vi "Test Set Subpanels-- Paths Array.vi"(8 "error in":errorcluster) -> (0 "error out":errorcluster)   [LabVIEW 2020]
uses:
  Maui 2.0/Maui 2.0.lvclass
  C:/Program Files (x86)/National Instruments/LabVIEW 2020/vi.lib/JKI/JKI SMO/SMO/SMO.lvclass
  <vilib>/addons/_JKI Toolkits/Caraya/classes/Assert/Assert True.vi
  <vilib>/JKI/JKI SMO/SMO/SMO.lvclass
  <vilib>/addons/_JKI Toolkits/Caraya/classes/Test/Test.lvclass
  <vilib>/addons/_JKI Toolkits/Caraya/classes/Assert/Assert.lvclass
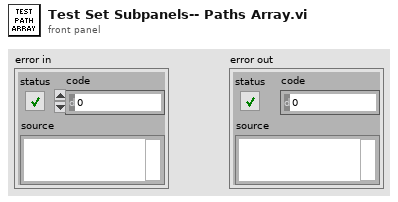
[diagram p1: front panel]
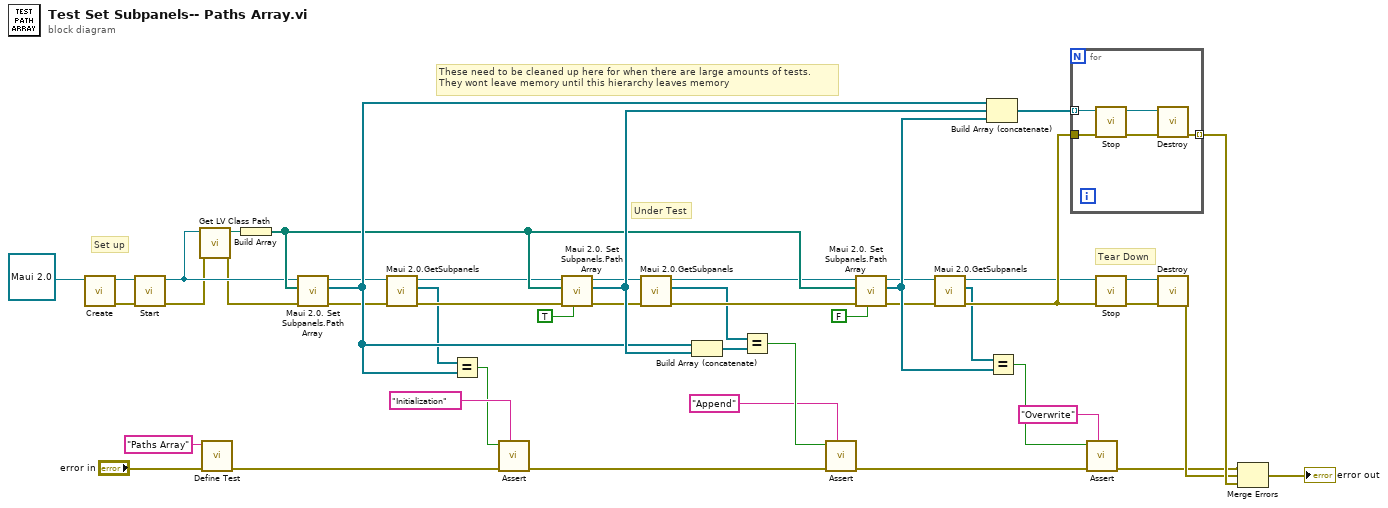
[diagram p0: block diagram]
diagram:
  # "These need to be cleaned up here for when there are large amounts of tests.\nThey wont leave memory until this hierarchy leaves memory"
  # "Tear Down"
  # "Set up"
  # "Under Test"
  n1 = call <vilib>:"Create.vi"("SMO"=refnum<class "Maui 2.0.lvclass"> refnum ("Maui 2.0.lvclass")) -> ("error out"=w3:errorcluster, "SMO out"=w2:refnum<class "Maui 2.0.lvclass">)  [unwired: 8 in, 1 out]
  n2 = call <vilib>:"Start.vi"("error in (no error)"=w3, "SMO"=w2) -> ("error out"=w13:errorcluster, "SMO out"=w15:refnum<class "Maui 2.0.lvclass">)  [unwired: 8 in]
  n3 = call <vilib>:"Get LV Class Path.vi"("error in (no error)"=w13, "object"=w15) -> ("error out"=w14:errorcluster, "class path"=w12:path)  [unwired: 8 in]
  n4 = call <vilib>:"Define Test.vi"("error in (no error)"="error in", "Label (VI Title)"="Paths Array") -> ("error out"=w41:errorcluster)  [unwired: 9 in]
  n5 = Build Array(w12) -> (w31:path[])
  n6 = call-dynamic "Maui 2.0. Set Subpanels.Path Array.vi"("error in (no error)"=w14, "Subpanel List"=w31, "Maui 2.0 in"=w15) -> ("error out"=w5:errorcluster, "Subpanels"=w42:refnum<class "SMO.lvclass">[], "Maui 2.0 out"=w4:refnum<class "Maui 2.0.lvclass">)  [unwired: 6 in]
  n7 = call "Maui 2.0.GetSubpanels.vi"("error in (no error)"=w5, "Maui 2.0"=w4) -> ("error out"=w18:errorcluster, "Subpanels"=w6:refnum<class "SMO.lvclass">[], "Maui 2.0 out"=w17:refnum<class "Maui 2.0.lvclass">)  [unwired: 7 in]
  n8 = Equal?(x=w6, y=w42) -> (x = y?=w10:bool)
  n9 = call-poly <vilib>:"Assert.vi"("Label"="Initialization", "error in (no error)"=w41, "True?"=w10) -> ("error out"=w33:errorcluster)  [unwired: 8 in]
  n10 = call-dynamic "Maui 2.0. Set Subpanels.Path Array.vi"("Append (F)"=TRUE, "error in (no error)"=w18, "Subpanel List"=w31, "Maui 2.0 in"=w17) -> ("error out"=w20:errorcluster, "Subpanels"=w43:refnum<class "SMO.lvclass">[], "Maui 2.0 out"=w19:refnum<class "Maui 2.0.lvclass">)  [unwired: 5 in]
  n11 = call "Maui 2.0.GetSubpanels.vi"("error in (no error)"=w20, "Maui 2.0"=w19) -> ("error out"=w30:errorcluster, "Subpanels"=w21:refnum<class "SMO.lvclass">[], "Maui 2.0 out"=w28:refnum<class "Maui 2.0.lvclass">)  [unwired: 7 in]
  n12 = Build Array (concatenate)(w42, w43) -> (w22:refnum<class "SMO.lvclass">[])
  n13 = Equal?(x=w21, y=w22) -> (x = y?=w25:bool)
  n14 = call-poly <vilib>:"Assert.vi"("Label"="Append", "error in (no error)"=w33, "True?"=w25) -> ("error out"=w34:errorcluster)  [unwired: 8 in]
  n15 = call-dynamic "Maui 2.0. Set Subpanels.Path Array.vi"("Append (F)"=FALSE, "error in (no error)"=w30, "Subpanel List"=w31, "Maui 2.0 in"=w28) -> ("error out"=w26:errorcluster, "Subpanels"=w44:refnum<class "SMO.lvclass">[], "Maui 2.0 out"=w27:refnum<class "Maui 2.0.lvclass">)  [unwired: 5 in]
  n16 = call "Maui 2.0.GetSubpanels.vi"("error in (no error)"=w26, "Maui 2.0"=w27) -> ("error out"=w46:errorcluster, "Subpanels"=w35:refnum<class "SMO.lvclass">[], "Maui 2.0 out"=w29:refnum<class "Maui 2.0.lvclass">)  [unwired: 7 in]
  n17 = Build Array (concatenate)(w42, w43, w44) -> (w45:refnum<class "SMO.lvclass">[])
  n18 = Equal?(x=w35, y=w44) -> (x = y?=w36:bool)
  n19 = for {
    tunnel: w45 -> [w50] mode=indexing
    tunnel: w46 -> [w49]
    tunnel: [w48] -> w47 mode=indexing
    n20 = call <vilib>:"Stop.vi"("error in (no error)"=w49, "SMO"=w50) -> ("error out"=w52:errorcluster, "SMO out"=w51:refnum<class "SMO.lvclass">)  [unwired: 8 in]
    n21 = call <vilib>:"Destroy.vi"("error in (no error)"=w52, "SMO"=w51) -> ("error out"=w48:errorcluster)  [unwired: 9 in]
  }
  n22 = call-poly <vilib>:"Assert.vi"("Label"="Overwrite", "error in (no error)"=w34, "True?"=w36) -> ("error out"=w38:errorcluster)  [unwired: 8 in]
  n23 = call <vilib>:"Stop.vi"("error in (no error)"=w46, "SMO"=w29) -> ("error out"=w8:errorcluster, "SMO out"=w7:refnum<class "Maui 2.0.lvclass">)  [unwired: 8 in]
  n24 = call <vilib>:"Destroy.vi"("error in (no error)"=w8, "SMO"=w7) -> ("error out"=w39:errorcluster)  [unwired: 9 in]
  n25 = Merge Errors(w38, w39, w47) -> (→"error out":errorcluster)
